vi "TSM SSC Digital Abort.vi"(0 "Digital TSM In":T1, 11 "error in":errorcluster) -> (4 "Digital TSM out":T1, 15 "error out":errorcluster)   [LabVIEW 2019]
doc: "Stops bursting the pattern on the specified pin(s) or pin group(s)."
uses:
  TSM/TSM SSC Digital.ctl
  <vilib>/NI_TestStand_SemiconductorModule/NI_TestStand_Semiconductor_Module.lvlibp/PinMap/Digital Pattern/PinQueryContext/DigitalPatternPinQueryContext.lvclass
  SSC Digital/SSC Digital.ctl
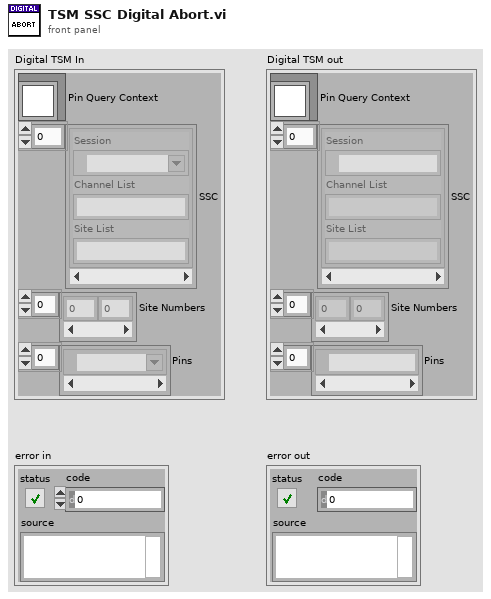
[diagram p1: front panel]
types:
  T1 = typedef "TSM SSC Digital.ctl" = cluster{"Pin Query Context":refnum<class "DigitalPatternPinQueryContext.lvclass">, "SSC":T2[], "Site Numbers":i32[], "Pins":tag[]}
  T2 = typedef "SSC Digital.ctl" = cluster{"Session":refnum<k15>, "Channel List":string, "Site List":string}
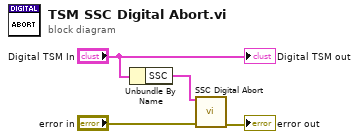
[diagram p0: block diagram]
diagram:
  n1 = Unbundle By Name("Digital TSM In") -> ("SSC"=w2:T2[])
  n2 = call "SSC Digital Abort.vi"("Digital SSC in"=w2, "error in"="error in") -> ("error out"=→"error out":errorcluster)  [unwired: 12 in, 1 out]
  "Digital TSM out" <- "Digital TSM In"
